vi "Example_BrainStemNetworking.vi"() -> ()   [LabVIEW 2021, in "BrainStem2_LabVIEW_Library.lvlib"]
uses:
  BrainStem2_LabVIEW_Library.lvlib
panel:
  out "LED 2":bool
  out "LED":bool
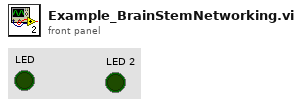
[diagram p1: front panel]
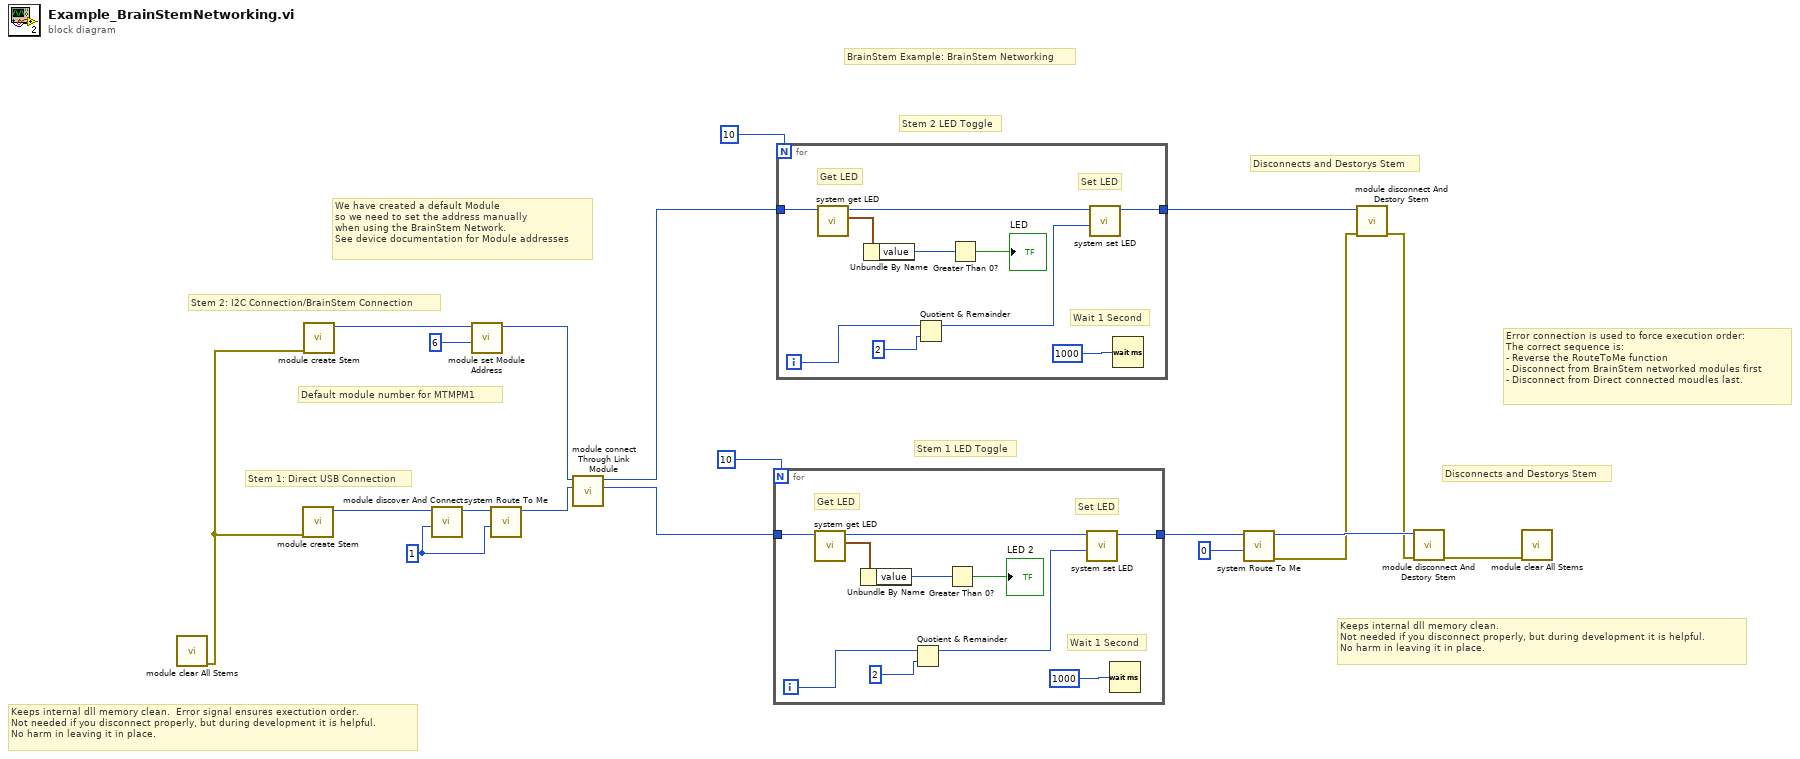
[diagram p0: block diagram]
diagram:
  w17 = 1
  # "Default module number for MTMPM1"
  # "Keeps internal dll memory clean. \nNot needed if you disconnect properly, but during development it is helpful. \nNo harm in leaving it in place."
  # "Keeps internal dll memory clean.  Error signal ensures exectution order.\nNot needed if you disconnect properly, but during development it is helpful. \nNo harm in leaving it in place."
  # "Stem 2 LED Toggle"
  # "Stem 1 LED Toggle"
  # "Stem 1: Direct USB Connection"
  # "Stem 2: I2C Connection/BrainStem Connection"
  # "We have created a default Module\nso we need to set the address manually\nwhen using the BrainStem Network.\nSee device documentation for Module addresses"
  # "Error connection is used to force execution order:\nThe correct sequence is:\n- Reverse the RouteToMe function\n- Disconnect from BrainStem networked modules first\n- Disconnect from Direct connected moudles last."
  # "Disconnects and Destorys Stem"
  # "BrainStem Example: BrainStem Networking"
  # "Disconnects and Destorys Stem"
  n1 = call "module clear All Stems.vi"() -> ("error out"=w4:errorcluster)  [unwired: 11 in]
  n2 = call "module create Stem.vi"("error in (no error)"=w4) -> ("id out"=w12:u32)  [unwired: 8 in, 2 out]
  n3 = call "module create Stem.vi"("error in (no error)"=w4) -> ("id out"=w8:u32)  [unwired: 8 in, 2 out]
  n4 = call "module discover And Connect.vi"("transport"=w17, "id"=w12) -> ("id out"=w11:u32)  [unwired: 7 in, 2 out]
  n5 = call "module set Module Address.vi"("address"=6, "id"=w8) -> ("id out"=w9:u32)  [unwired: 7 in, 2 out]
  n6 = call "system Route To Me.vi"("bOn"=w17, "id"=w11) -> ("id out"=w10:u32)  [unwired: 7 in, 2 out]
  n7 = call "module connect Through Link Module.vi"("id_linkStem"=w10, "id"=w9) -> ("id_linkStem out"=w5:u32, "id out"=w6:u32)  [unwired: 6 in, 2 out]
  n8 = for {
    N: 10 -> [_]
    tunnel: w5 -> [w29]
    tunnel: [w27] -> w13
    i -> [w22]
    # "Wait 1 Second"
    # "Set LED"
    # "Get LED"
    n9 = call "system get LED.vi"("id"=w29) -> ("result out"=w26:cluster{"value":i32, "error":i32}, "id out"=w28:u32)  [unwired: 8 in, 1 out]
    n10 = Unbundle By Name(w26) -> ("value"=w24:i32)
    n11 = Quotient & Remainder(x=w22, y=2) -> (x-y*floor(x/y)=w21:i32)  [unwired: 1 out]
    n12 = Greater Than 0?(x=w24) -> (x > 0?=→"LED 2":bool)
    n13 = call "system set LED.vi"("bOn"=w21, "id"=w28) -> ("id out"=w27:u32)  [unwired: 7 in, 2 out]
    n14 = Wait (ms)(milliseconds to wait=1000) -> ()  [unwired: 1 out]
  }
  n15 = for {
    N: 10 -> [_]
    tunnel: w6 -> [w39]
    tunnel: [w37] -> w14
    i -> [w32]
    # "Wait 1 Second"
    # "Set LED"
    # "Get LED"
    n16 = call "system get LED.vi"("id"=w39) -> ("result out"=w36:cluster{"value":i32, "error":i32}, "id out"=w38:u32)  [unwired: 8 in, 1 out]
    n17 = Unbundle By Name(w36) -> ("value"=w34:i32)
    n18 = Quotient & Remainder(x=w32, y=2) -> (x-y*floor(x/y)=w31:i32)  [unwired: 1 out]
    n19 = Greater Than 0?(x=w34) -> (x > 0?=→"LED":bool)
    n20 = call "system set LED.vi"("bOn"=w31, "id"=w38) -> ("id out"=w37:u32)  [unwired: 7 in, 2 out]
    n21 = Wait (ms)(milliseconds to wait=1000) -> ()  [unwired: 1 out]
  }
  n22 = call "system Route To Me.vi"("bOn"=0, "id"=w13) -> ("error out"=w2:errorcluster, "id out"=w15:u32)  [unwired: 7 in, 1 out]
  n23 = call "module disconnect And Destory Stem.vi"("error in (no error)"=w2, "id"=w14) -> ("error out"=w3:errorcluster)  [unwired: 7 in, 2 out]
  n24 = call "module disconnect And Destory Stem.vi"("error in (no error)"=w3, "id"=w15) -> ("error out"=w1:errorcluster)  [unwired: 7 in, 2 out]
  n25 = call "module clear All Stems.vi"("error in (no error)"=w1) -> ()  [unwired: 10 in, 1 out]
